vi "subVI QCam Calculate Exposure Ratios.vi"(2 "exposure Blue":dbl, 3 "exposure Red":dbl, 4 "exposure":dbl) -> (0 "Ratio BlueGreen":dbl, 1 "Ratio RedGreen":dbl)   [LabVIEW 2012]
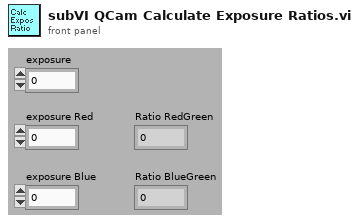
[diagram p1: front panel]
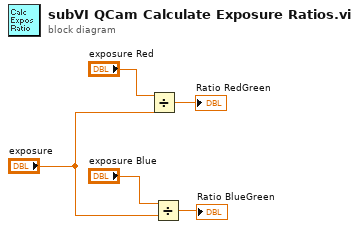
[diagram p0: block diagram]
diagram:
  n1 = Divide(x="exposure Red", y="exposure") -> (x/y=→"Ratio RedGreen":dbl)
  n2 = Divide(x="exposure Blue", y="exposure") -> (x/y=→"Ratio BlueGreen":dbl)
